vi "Periodic Tasks.vi"(8 "error in":errorcluster) -> ()   [LabVIEW 2014]
doc: "This VI runs in parallel to other tasks. It can contain as many user-defined periodic loops as you need. These can carry out PID or other sorts of timed response."
uses:
  <vilib>/Rock Robotics/WPI/Solenoid/WPI_SolenoidValue.ctl
  <vilib>/Rock Robotics/WPI/Joystick/WPI_JoystickGetSetRefNum.vi
  Robot Global Data.vi
  <vilib>/Rock Robotics/Network Tables/SD Write Boolean.vi
  <vilib>/Rock Robotics/Network Tables/SD Write Number.vi
  <vilib>/Rock Robotics/WPI/RobotDrive/WPI_RobotDriveGetSetRefNum.vi
  <vilib>/Rock Robotics/WPI/Solenoid/WPI_SolenoidSetEnum.vi
panel:
  out "pnumatics button 2":bool
  in  "Stopper Motor Speed Up":dbl(slide)=0.6 min=-1.0 max=1.0 step=0.05 scale=0.0..1.0 scale format="%#.3f"
  in  "Stopper Motor Speed Down":dbl(slide)=0.2 min=-1.0 max=1.0 step=0.05 scale=0.0..1.0 scale format="%#.3f"
  out "Actual Stopper Motor Speed":dbl
  out "Lifting Motor Speed Up":dbl
  out "Mode":bool
  out "Actual Lifting Motor Speed":dbl format="%#_13g"
  out "Trigger Switch Activated":bool=TRUE
  out "Upper Switch Activated":bool=TRUE
  out "Lower Switch Activated":bool=TRUE
  out "Accelerometer Chart":cluster{"X-Axis":dbl, "Y-Axis":dbl}(graph)
  out "X Acceleration":dbl format="%#_13g"
  out "Y Acceleration":dbl format="%#_13g"
  out "Degrees of Rotation":dbl format="%#_13g"
  out "pnumatics button":bool
  out "L":bool
  out "U":bool
  out "T":bool
  out "Running":bool
  out "Direction":bool
  in  "Lifting Motor Speed Down":dbl(slide)=0.39999999999999997 min=-1.0 max=1.0 step=0.05 scale=0.0..1.0 scale format="%#.3f"
  # "STOPPER\nMOTOR PANEL"
  # "GANTRY LIFT\nMOTOR PANEL"
  # "INDICATORS"
  # "LOGIC"
  # "CONTROLS"
  # "CONTROLS"
  # "INDICATORS"
  # "ACCELEROMETER\nPANEL"
  # "PNEUMATICS\nPANEL"
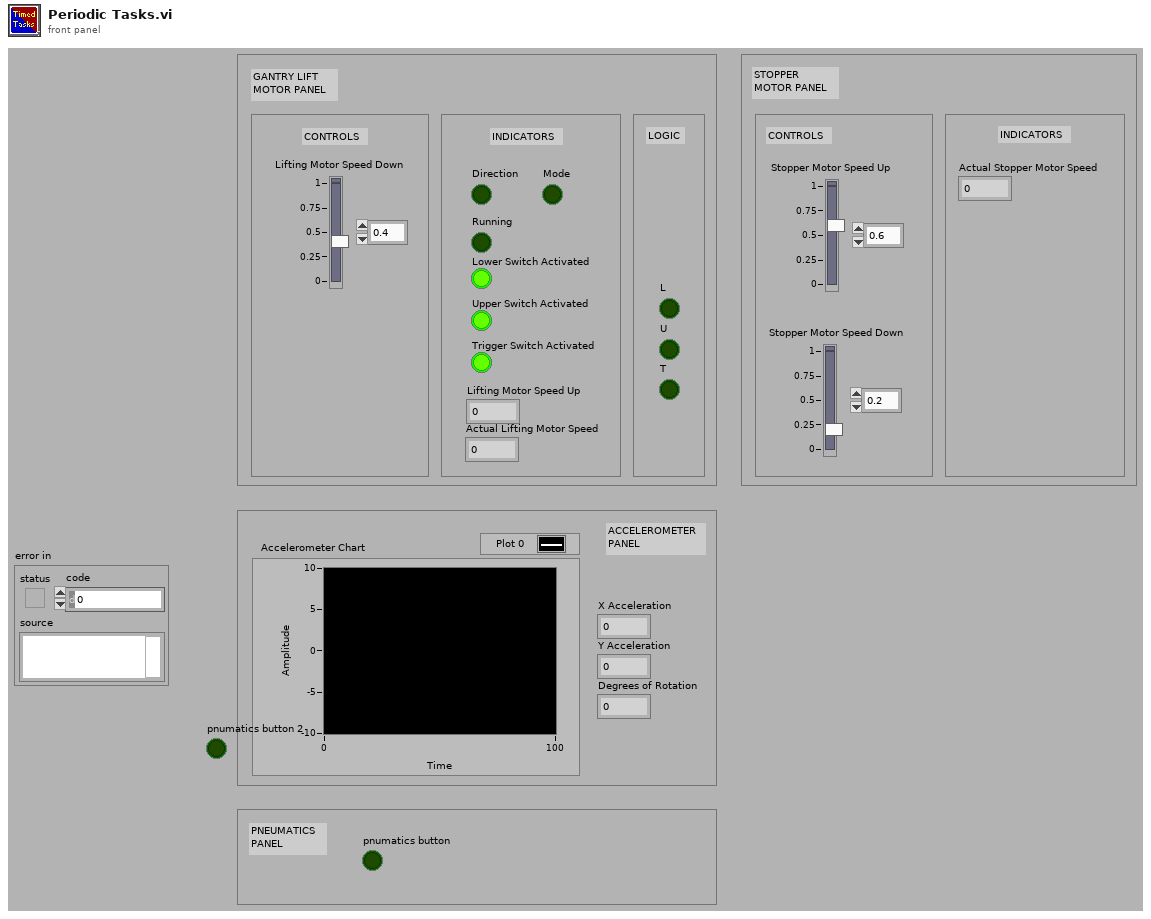
[diagram p1: front panel]
types:
  T1 = typedef "WPI_SolenoidValue.ctl" = enum16{"Off", "On", "Forward", "Reverse"}
  T2 = typedef "WPI_JoystickDevRef.ctl" = cluster{"Device":T3}
  T3 = typedef "WPI_JoystickDeviceEnum.ctl" = enum16{"USB 0", "USB 1", "USB 2", "USB 3", "USB 4", "USB 5"}
  T4 = typedef "WPI_SolenoidDevRef.ctl" = cluster{"DevStatus":errorcluster, "Pneumatics Control Module":u8, "Forward Solenoid Channel":T5, "Reverse Solenoid Channel":T5}
  T5 = typedef "WPI_SolenoidChannel.ctl" = enum8{"Solenoid 0", "Solenoid 1", "Solenoid 2", "Solenoid 3", "Solenoid 4", "Solenoid 5", "Solenoid 6", "Solenoid 7", "Invalid"}
  T6 = cluster{"JoystickDevRef":T2, "SolenoidDevRef":T4}
  T7 = typedef "WPI_AccelerometerDevRef.ctl" = cluster{"DevStatus":errorcluster, "Controller":T8, "Scaling":T9, "Analog Channels":T10, "I2C Bus":T12, "SPI Bus":T13, "Accel Range":T14, "ADXL345 Axes":T15, "Handle":i32, "Device Address":u8, "Accel Type":enum16{"Analog", "ADXL345 I2C", "ADXL345 SPI", "Internal"}}
  T8 = typedef "FPGA_TypedefAnalogModule.ctl" = enum16{"Controller 1"}
  T9 = typedef "WPI_AccelerometerScaling.ctl" = cluster{"Gain (VoltsPerG)":dbl, "Center Voltage":dbl}
  T10 = typedef "WPI_AccelerometerAnalogChannels.ctl" = cluster{"X-Axis":T11, "Y-Axis":T11, "Z-Axis":T11}
  T11 = typedef "FPGA_AIChannel.ctl" = enum8{"AI 0", "AI 1", "AI 2", "AI 3", "AI MXP 0", "AI MXP 1", "AI MXP 2", "AI MXP 3", "Invalid"}
  T12 = typedef "i2c_bus.ctl" = enum16{"I2C On-Board", "I2C MXP", "Invalid"}
  T13 = typedef "spi_bus.ctl" = enum16{"SPI On-Board, CS0", "SPI On-Board, CS1", "SPI On-Board, CS2", "SPI On-Board, CS3", "SPI MXP", "Invalid"}
  T14 = typedef "ADXL345 Range.ctl" = u8
  T15 = typedef "WPI_AccelerometerADXL345 Axes.ctl" = cluster{"X-Axis":bool, "Y-Axis":bool, "Z-Axis":bool}
  T16 = cluster{"X-Axis":dbl, "Y-Axis":dbl, "Z-Axis":dbl}
  T17 = typedef "WPI_MotorControlDeviceRef.ctl" = cluster{"DeviceStatus":errorcluster, "Type":T18, "PWM":cluster{"Controller":T19, "PWM Channel":T20, "DeadBand":T21}, "CAN":cluster{"Device Number":u8, "Control Mode":T22, "Semaphore":T23, "Max Vout":dbl, "TalonSRX Control Mode":T24}, "Invert":bool, "TransformRef":T25, "InvTransformRef":T25}
  T18 = typedef "WPI_MotorControlType.ctl" = enum16{"PWM", "CAN", "CANTalonSRX"}
  T19 = typedef "FPGA_TypedefDigitalModule.ctl" = enum16{"Controller 1"}
  T20 = typedef "FPGA_DIOPWMChannel.ctl" = enum8{"PWM 0", "PWM 1", "PWM 2", "PWM 3", "PWM 4", "PWM 5", "PWM 6", "PWM 7", "PWM 8", "PWM 9", "PWM MXP 0", "PWM MXP 1", "PWM MXP 2", "PWM MXP 3", "PWM MXP 4", "PWM MXP 5", "PWM MXP 6", "PWM MXP 7", "PWM MXP 8", "PWM MXP 9", "Invalid"}
  T21 = typedef "WPI_PWMDeadband.ctl" = cluster{"Name":string, "maxPositivePwm":i32, "minPositivePwm":i32, "centerPwm":i32, "maxNegativePwm":i32, "minNegativePwm":i32, "angularRange":u16}
  T22 = typedef "WPI_CANJaguar_ControlMode.ctl" = enum8{"Percent VBus", "Current", "Speed", "Position", "Voltage"}
  T23 = typedef "Semaphore RefNum" = refnum<k1>
  T24 = typedef "WPI_CANTalonSRX_APIControlMode.ctl" = enum8{"Percent VBus", "Speed", "Position", "Slave", "Unchanged / Invalid"}
  T25 = typedef "WPI_PWMTransform_ConPane.ctl" = refnum<vi>
  T26 = typedef "WPI_DigitalInputDevRef.ctl" = cluster{"DevStatus":errorcluster, "DIO Channel":T27, "Controller":T19}
  T27 = typedef "FPGA_DIOChannel.ctl" = enum8{"DIO 0", "DIO 1", "DIO 2", "DIO 3", "DIO 4", "DIO 5", "DIO 6", "DIO 7", "DIO 8", "DIO 9", "DIO MXP 0", "DIO MXP 1", "DIO MXP 2", "DIO MXP 3", "DIO MXP 4", "DIO MXP 5", "DIO MXP 6", "DIO MXP 7", "DIO MXP 8", "DIO MXP 9", "DIO MXP 10", "DIO MXP 11", "DIO MXP 12", "DIO MXP 13", "DIO MXP 14", "DIO MXP 15", "Invalid"}
  T28 = cluster{"JoystickDevRef":T2, "MotorControlDevRef":T17}
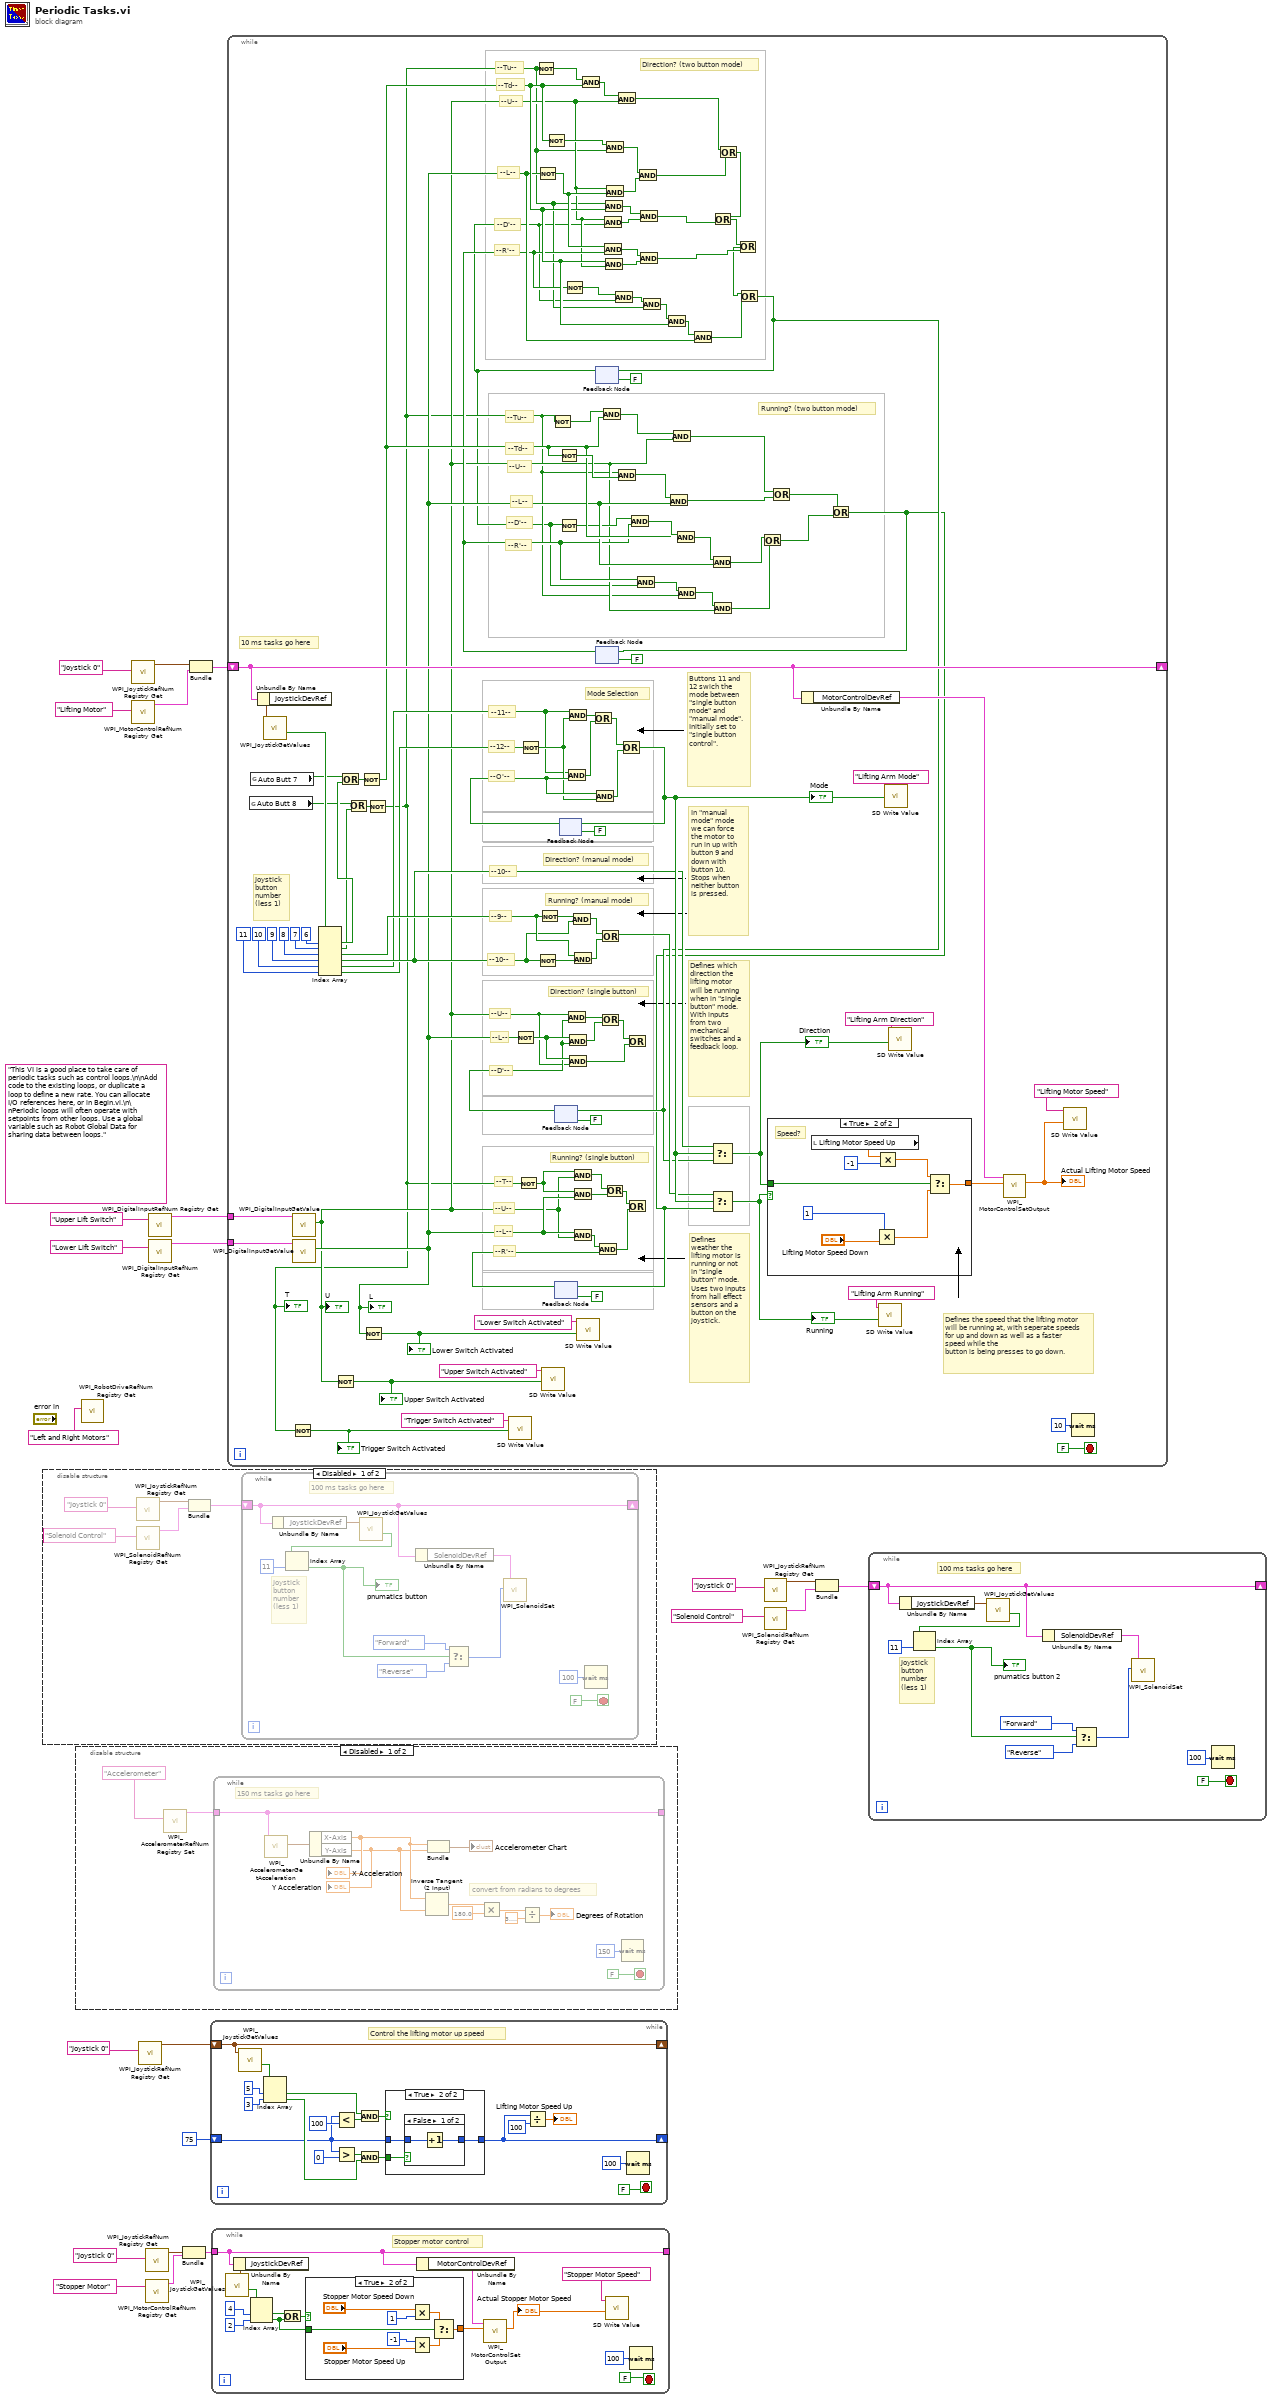
[diagram p0: block diagram]
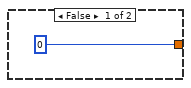
[diagram p2: hidden frame]
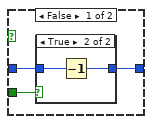
[diagram p3: hidden frame]
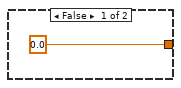
[diagram p8: hidden frame]
diagram:
  (unwired) "This VI is a good place to take care of periodic tasks such as control loops.\n\nAdd code to the existing loops, or duplicate a loop to define a new rate. You can allocate I/O references here, or in Begin.vi.\n\nPeriodic loops will often operate with setpoints from other loops. Use a global variable such as Robot Global Data for sharing data between loops."
  n1 = disable-structure shown="Disabled" {
    frame Disabled {
      n2 = call <vilib>:"WPI_JoystickRefNum Registry Get.vi"("refnum name"="Joystick 0") -> ("JoystickDevRef"=w26:T2)  [unwired: 1 in, 9 out]
      n3 = call <vilib>:"WPI_SolenoidRefNum Registry Get.vi"("refnum name"="Solenoid Control") -> ("SolenoidDevRef"=w25:T4)  [unwired: 9 in, 1 out]
      n4 = Bundle("JoystickDevRef"=w26, "SolenoidDevRef"=w25) -> (w24:T6)  [unwired: 1 out]
      n5 = while {
        shift-right: [w34] -> _
        shift-left: w24 -> [w34]
        stop <- FALSE stop-if-true
        # "Joystick button number (less 1)"
        # "100 ms tasks go here"
        n6 = Unbundle By Name(w34) -> ("JoystickDevRef"=w37:T2)
        n7 = call <vilib>:"WPI_JoystickGetValues.vi"("JoystickDevRef"=w37) -> ("Buttons"=w36:bool[])  [unwired: 6 in, 4 out]
        n8 = Index Array(array=w36, index=11) -> (element=w32:bool)
        "pnumatics button" <- w32
        n9 = Unbundle By Name(w34) -> ("SolenoidDevRef"=w33:T4)
        n10 = Select(t=WPI_SolenoidValue."Forward" ("Relay Value"), s=w32, f=WPI_SolenoidValue."Reverse" ("Relay Value")) -> (s? t:f=w29:T1)
        n11 = call-poly <vilib>:"WPI_SolenoidSet.vi"("Value"=w29, "SolenoidDevRef"=w33) -> ()  [unwired: 8 in, 2 out]
        n12 = Wait (ms)(milliseconds to wait=u32 100) -> ()  [unwired: 1 out]
      }
    }
    frame Enabled {
    }
  }
  n13 = disable-structure shown="Disabled" {
    frame Disabled {
      n14 = call <vilib>:"WPI_AccelerometerRefNum Registry Set.vi"("refnum name"="Accelerometer") -> ("AccelerometerDevRef"=w40:T7)  [unwired: 9 in, 1 out]
      n15 = while {
        tunnel: [w51] -> _
        tunnel: w40 -> [w51]
        stop <- FALSE stop-if-true
        # "convert from radians to degrees"
        # "150 ms tasks go here"
        n16 = call <vilib>:"WPI_AccelerometerGetAcceleration.vi"("AccelerometerDevRef"=w51) -> ("Accelerations"=w46:T16)  [unwired: 8 in, 2 out]
        n17 = Unbundle By Name(w46) -> ("X-Axis"=w44:dbl, "Y-Axis"=w43:dbl)
        "X Acceleration" <- w44
        "Y Acceleration" <- w43
        n18 = Inverse Tangent (2 Input)(1:w43, 2:w44) -> (0:w47:dbl)
        n19 = Bundle("X-Axis"=w44, "Y-Axis"=w43) -> (→"Accelerometer Chart":cluster{"X-Axis":dbl, "Y-Axis":dbl})  [unwired: 1 in]
        n20 = Multiply(x=w47, y=180.0) -> (x*y=w49:dbl)
        n21 = Divide(x=w49, y=3.141592653589793) -> (x/y=→"Degrees of Rotation":dbl)
        n22 = Wait (ms)(milliseconds to wait=u32 150) -> ()  [unwired: 1 out]
      }
    }
    frame Enabled {
    }
  }
  n23 = call <vilib>:"WPI_RobotDriveRefNum Registry Get.vi"("refnum name"="Left and Right Motors") -> ()  [unwired: 1 in, 10 out]
  n24 = call <vilib>:"WPI_JoystickRefNum Registry Get.vi"("refnum name"="Joystick 0") -> ("JoystickDevRef"=w19:T2)  [unwired: 1 in, 9 out]
  n25 = call <vilib>:"WPI_MotorControlRefNum Registry Get.vi"("refnum name"="Lifting Motor") -> ("MotorControlDevRef"=w15:T17)  [unwired: 9 in, 1 out]
  n26 = call <vilib>:"WPI_JoystickRefNum Registry Get.vi"("refnum name"="Joystick 0") -> ("JoystickDevRef"=w6:T2)  [unwired: 1 in, 9 out]
  n27 = call <vilib>:"WPI_JoystickRefNum Registry Get.vi"("refnum name"="Joystick 0") -> ("JoystickDevRef"=w10:T2)  [unwired: 1 in, 9 out]
  n28 = call <vilib>:"WPI_MotorControlRefNum Registry Get.vi"("refnum name"="Stopper Motor") -> ("MotorControlDevRef"=w9:T17)  [unwired: 9 in, 1 out]
  n29 = call <vilib>:"WPI_DigitalInputRefNum Registry Get.vi"("refnum name"="Upper Lift Switch") -> ("DigitalInputDevRef"=w17:T26)  [unwired: 9 in, 1 out]
  n30 = call <vilib>:"WPI_DigitalInputRefNum Registry Get.vi"("refnum name"="Lower Lift Switch") -> ("DigitalInputDevRef"=w16:T26)  [unwired: 9 in, 1 out]
  n31 = Bundle("JoystickDevRef"=w10, "MotorControlDevRef"=w9) -> (w8:T28)  [unwired: 1 in]
  n32 = Bundle("JoystickDevRef"=w19, "MotorControlDevRef"=w15) -> (w22:T28)  [unwired: 1 out]
  n33 = while {
    shift-right: [w64] -> _
    shift-left: 75 -> [w54]
    shift-right: [w56] -> _
    shift-left: w6 -> [w56]
    stop <- FALSE stop-if-true
    # "Control the lifting motor up speed"
    n34 = call <vilib>:"WPI_JoystickGetValues.vi"("JoystickDevRef"=w56) -> ("Buttons"=w62:bool[])  [unwired: 6 in, 4 out]
    n35 = Index Array(array=w62, index #1=5, index #2=3) -> (element #1=w59:bool, element #2=w58:bool)
    n36 = Less?(x=w54, y=100) -> (x < y?=w68:bool)
    n37 = Greater?(x=w54, y=0) -> (0:w67:bool)
    n38 = And(x=w59, y=w68) -> (x .and. y?=w66:bool)
    n39 = And(x=w67, y=w58) -> (x .and. y?=w65:bool)
    n40 = case shown="True" w66 {
      tunnel: w65 -> [w74 w80]
      tunnel: w54 -> [w73 w79]
      tunnel: [w72 w78] -> w64
      frame False {
        n41 = case shown="True" w74 {
          tunnel: w73 -> [w75 w77]
          tunnel: [w75 w76] -> w72
          frame False {
          }
          frame True {
            n42 = Decrement(x=w77) -> (x-1=w76:i32)
          }
        }
      }
      frame True {
        n43 = case shown="False" w80 {
          tunnel: w79 -> [w82 w83]
          tunnel: [w81 w83] -> w78
          frame False {
            n44 = Increment(x=w82) -> (x+1=w81:i32)
          }
          frame True {
          }
        }
      }
    }
    n45 = Divide(x=w64, y=100) -> (x/y=→"Lifting Motor Speed Up":dbl)
    n46 = Wait (ms)(milliseconds to wait=u32 100) -> ()  [unwired: 1 out]
  }
  n47 = while {
    tunnel: w8 -> [w88]
    tunnel: [w88] -> _
    stop <- FALSE stop-if-true
    # "Stopper motor control"
    n48 = Unbundle By Name(w88) -> ("JoystickDevRef"=w89:T2)
    n49 = call <vilib>:"WPI_JoystickGetValues.vi"("JoystickDevRef"=w89) -> ("Buttons"=w95:bool[])  [unwired: 6 in, 4 out]
    n50 = Index Array(array=w95, index #1=4, index #2=2) -> (element #1=w92:bool, element #2=w90:bool)
    n51 = Or(x=w92, y=w90) -> (x .or. y?=w91:bool)
    n52 = case shown="True" w91 {
      tunnel: w90 -> [_ w106]
      tunnel: [0 w104] -> w86
      frame False {
      }
      frame True {
        n53 = Multiply(x="Stopper Motor Speed Down", y=1) -> (x*y=w105:dbl)
        n54 = Multiply(x=-1, y="Stopper Motor Speed Up") -> (x*y=w101:dbl)
        n55 = Select(t=w105, s=w106, f=w101) -> (s? t:f=w104:dbl)
      }
    }
    n56 = Unbundle By Name(w88) -> ("MotorControlDevRef"=w87:T17)
    n57 = call <vilib>:"WPI_MotorControlSetOutput.vi"("Output"=w86, "MotorControlDevRef"=w87) -> ("Motor Output"=w84:dbl)  [unwired: 7 in, 2 out]
    "Actual Stopper Motor Speed" <- w84
    n58 = call-poly <vilib>:"SD Write Value.vi"("Numeric"=w84, "Name"="Stopper Motor Speed" ("refnum name")) -> ()  [unwired: 8 in, 2 out]
    n59 = Wait (ms)(milliseconds to wait=u32 100) -> ()  [unwired: 1 out]
  }
  n60 = while {
    shift-right: [w213] -> _
    shift-left: w22 -> [w213]
    tunnel: w17 -> [w217]
    tunnel: w16 -> [w215]
    stop <- FALSE stop-if-true
    # "Running? (two button mode)"
    # "Direction? (two button mode)"
    # "--R'--"
    # "--D'--"
    # "--L--"
    # "--U--"
    # "--Td--"
    # "--Tu--"
    # "--D'--"
    # "--R'--"
    # "--L--"
    # "--U--"
    # "--Td--"
    # "--Tu--"
    # "--10--"
    # "Direction? (manual mode)"
    # "--R'--"
    # "Running? (manual mode)"
    # "--O'--"
    # "Defines the speed that the lifting motor will be running at, with seperate speeds for up and down as well as a faster speed while the \nbutton is being presses to go down."
    # "Defines weather the lifting motor is running or not in \"single button\" mode. Uses two inputs from hall effect sensors and a button on the joystick."
    # "Defines which direction the lifting motor will be running when in \"single button\" mode. With inputs from two mechanical switches and a feedback loop."
    # "In \"manual mode\" mode we can force the motor to run in up with button 9 and down with button 10. Stops when neither button is pressed."
    # "Buttons 11 and 12 swich the mode between  \"single button mode\" and \"manual mode\". Initially set to \"single button control\"."
    # "--12--"
    # "--11--"
    # "--10--"
    # "--9--"
    # "Mode Selection"
    # "Joystick button number (less 1)"
    # "--U--"
    # "--L--"
    # "--T--"
    # "--D'--"
    # "--U--"
    # "--L--"
    # "Direction? (single button)"
    # "Running? (single button)"
    # "10 ms tasks go here"
    n61 = global read "Robot Global Data.vi" "Auto Butt 8"() -> (w109:bool)
    n62 = global read "Robot Global Data.vi" "Auto Butt 7"() -> (w113:bool)
    n63 = Unbundle By Name(w213) -> ("JoystickDevRef"=w216:T2)
    n64 = call <vilib>:"WPI_JoystickGetValues.vi"("JoystickDevRef"=w216) -> ("Buttons"=w195:bool[])  [unwired: 6 in, 4 out]
    n65 = call <vilib>:"WPI_DigitalInputGetValue.vi"("DigitalInputDevRef"=w217) -> ("Value"=w125:bool)  [unwired: 8 in, 2 out]
    "U" <- w125
    n66 = call <vilib>:"WPI_DigitalInputGetValue.vi"("DigitalInputDevRef"=w215) -> ("Value"=w131:bool)  [unwired: 8 in, 2 out]
    "L" <- w131
    n67 = Index Array(array=w195, index #1=u32 6 ("milliseconds to wait"), index #2=u32 7 ("milliseconds to wait"), index #3=u32 8 ("milliseconds to wait"), index #4=u32 9 ("milliseconds to wait"), index #5=u32 10 ("milliseconds to wait"), index #6=u32 11 ("milliseconds to wait")) -> (element #1=w112:bool, element #2=w110:bool, element #3=w170:bool, element #4=w166:bool, element #5=w163:bool, element #6=w162:bool)
    n68 = Not(x=w125) -> (.not. x?=w202:bool)
    "Upper Switch Activated" <- w202
    n69 = Or(x=w113, y=w112) -> (x .or. y?=w111:bool)
    n70 = Or(x=w109, y=w110) -> (x .or. y?=w197:bool)
    n71 = Not(x=w111) -> (.not. x?=w133:bool)
    n72 = Not(x=w131) -> (.not. x?=w203:bool)
    "Lower Switch Activated" <- w203
    n73 = Not(x=w197) -> (.not. x?=w124:bool)
    "T" <- w124
    n74 = Not(x=w124) -> (.not. x?=w200:bool)
    "Trigger Switch Activated" <- w200
    n75 = call-poly <vilib>:"SD Write Value.vi"("Boolean"=w200, "Name"="Trigger Switch Activated" ("refnum name")) -> ()  [unwired: 8 in, 2 out]
    n76 = Not(x=w131) -> (.not. x?=w183:bool)
    n77 = Not(x=w124) -> (.not. x?=w186:bool)
    n78 = Not(x=w162) -> (.not. x?=w177:bool)
    n79 = Not(x=w124) -> (.not. x?=w160:bool)
    n80 = Not(x=w131) -> (.not. x?=w139:bool)
    n81 = Not(x=w166) -> (.not. x?=w171:bool)
    n82 = Not(x=w170) -> (.not. x?=w172:bool)
    n83 = call-poly <vilib>:"SD Write Value.vi"("Boolean"=w202, "Name"="Upper Switch Activated" ("refnum name")) -> ()  [unwired: 8 in, 2 out]
    n84 = Not(x=w133) -> (.not. x?=w157:bool)
    n85 = Not(x=w124) -> (.not. x?=w126:bool)
    n86 = feedback #1(FALSE) -> (w178:bool)
    n87 = feedback #2(FALSE) -> (w185:bool)
    n88 = Not(x=w133) -> (.not. x?=w135:bool)
    n89 = feedback #3(FALSE) -> (w190:bool)
    n90 = And(x=w163, y=w190) -> (x .and. y?=w193:bool)
    n91 = And(x=w125, y=w178) -> (x .and. y?=w181:bool)
    n92 = And(x=w163, y=w177) -> (x .and. y?=w194:bool)
    n93 = And(x=w183, y=w178) -> (x .and. y?=w180:bool)
    n94 = And(x=w183, y=w125) -> (x .and. y?=w179:bool)
    n95 = And(x=w172, y=w166) -> (x .and. y?=w169:bool)
    n96 = And(x=w170, y=w171) -> (x .and. y?=w168:bool)
    n97 = And(x=w186, y=w125) -> (x .and. y?=w208:bool)
    n98 = And(x=w186, y=w131) -> (x .and. y?=w207:bool)
    n99 = And(x=w131, y=w125) -> (x .and. y?=w187:bool)
    n100 = call-poly <vilib>:"SD Write Value.vi"("Boolean"=w203, "Name"="Lower Switch Activated" ("refnum name")) -> ()  [unwired: 8 in, 2 out]
    n101 = And(x=w160, y=w133) -> (x .and. y?=w158:bool)
    n102 = Or(x=w194, y=w193) -> (x .or. y?=w192:bool)
    n103 = And(x=w190, y=w177) -> (x .and. y?=w191:bool)
    n104 = feedback #4(FALSE) -> (w123:bool)
    n105 = Not(x=w123) -> (.not. x?=w127:bool)
    n106 = feedback #5(FALSE) -> (w128:bool)
    n107 = Not(x=w128) -> (.not. x?=w138:bool)
    n108 = And(x=w187, y=w185) -> (x .and. y?=w184:bool)
    n109 = Or(x=w169, y=w168) -> (x .or. y?=w167:bool)
    n110 = Or(x=w181, y=w180) -> (x .or. y?=w182:bool)
    n111 = And(x=w126, y=w133) -> (x .and. y?=w137:bool)
    n112 = And(x=w125, y=w123) -> (x .and. y?=w151:bool)
    n113 = And(x=w139, y=w128) -> (x .and. y?=w148:bool)
    n114 = And(x=w124, y=w133) -> (x .and. y?=w152:bool)
    n115 = And(x=w133, y=w125) -> (x .and. y?=w147:bool)
    n116 = And(x=w157, y=w124) -> (x .and. y?=w156:bool)
    n117 = And(x=w125, y=w139) -> (x .and. y?=w155:bool)
    n118 = Or(x=w208, y=w207) -> (x .or. y?=w206:bool)
    n119 = And(x=w138, y=w123) -> (x .and. y?=w144:bool)
    n120 = And(x=w158, y=w125) -> (x .and. y?=w116:bool)
    n121 = And(x=w124, y=w135) -> (x .and. y?=w136:bool)
    n122 = Or(x=w192, y=w191) -> (x .or. y?=w175:bool)
    "Mode" <- w175
    n123 = feedback-in #3(w175) -> ()
    n124 = Or(x=w182, y=w179) -> ()  [unwired: 1 out]
    n125 = Or(x=w206, y=w184) -> ()  [unwired: 1 out]
    n126 = And(x=w127, y=w128) -> (x .and. y?=w134:bool)
    n127 = And(x=w128, y=w123) -> (x .and. y?=w129:bool)
    n128 = And(x=w156, y=w155) -> (x .and. y?=w154:bool)
    n129 = And(x=w152, y=w151) -> (x .and. y?=w150:bool)
    n130 = And(x=w148, y=w147) -> (x .and. y?=w146:bool)
    n131 = And(x=w144, y=w124) -> (x .and. y?=w143:bool)
    n132 = And(x=w143, y=w133) -> (x .and. y?=w142:bool)
    n133 = And(x=w136, y=w131) -> (x .and. y?=w121:bool)
    n134 = And(x=w137, y=w125) -> (x .and. y?=w122:bool)
    n135 = And(x=w134, y=w133) -> (x .and. y?=w132:bool)
    n136 = And(x=w129, y=w124) -> (x .and. y?=w130:bool)
    n137 = And(x=w142, y=w131) -> (x .and. y?=w140:bool)
    n138 = And(x=w132, y=w131) -> (x .and. y?=w120:bool)
    n139 = And(x=w130, y=w125) -> (x .and. y?=w119:bool)
    n140 = Or(x=w116, y=w154) -> (x .or. y?=w161:bool)
    n141 = Or(x=w161, y=w150) -> (x .or. y?=w145:bool)
    n142 = Or(x=w145, y=w146) -> (x .or. y?=w141:bool)
    n143 = Or(x=w141, y=w140) -> (x .or. y?=w115:bool)
    n144 = feedback-in #1(w115) -> ()
    n145 = feedback-in #4(w115) -> ()
    n146 = Select(t=w166, s=w175, f=w115) -> (s? t:f=w174:bool)
    "Direction" <- w174
    n147 = Or(x=w120, y=w119) -> (x .or. y?=w117:bool)
    n148 = Or(x=w122, y=w121) -> (x .or. y?=w118:bool)
    n149 = Unbundle By Name(w213) -> ("MotorControlDevRef"=w212:T17)
    n150 = Or(x=w118, y=w117) -> (x .or. y?=w114:bool)
    n151 = feedback-in #2(w114) -> ()
    n152 = feedback-in #5(w114) -> ()
    n153 = Select(t=w167, s=w175, f=w114) -> (s? t:f=w173:bool)
    "Running" <- w173
    n154 = case shown="True" w173 {
      tunnel: w174 -> [_ w228]
      tunnel: [0.0 ("Throw Motor Speed (-1 to 1) 2") w227] -> w198
      frame False {
      }
      frame True {
        # "Speed?"
        n155 = local read "Lifting Motor Speed Up"() -> (w221:dbl)
        n156 = Multiply(x=1, y="Lifting Motor Speed Down") -> (x*y=w224:dbl)
        n157 = Multiply(x=w221, y=-1) -> (x*y=w225:dbl)
        n158 = Select(t=w225, s=w228, f=w224) -> (s? t:f=w227:dbl)
      }
    }
    n159 = call-poly <vilib>:"SD Write Value.vi"("Boolean"=w173, "Name"="Lifting Arm Running" ("refnum name")) -> ()  [unwired: 8 in, 2 out]
    n160 = call-poly <vilib>:"SD Write Value.vi"("Boolean"=w175, "Name"="Lifting Arm Mode" ("refnum name")) -> ()  [unwired: 8 in, 2 out]
    n161 = call-poly <vilib>:"SD Write Value.vi"("Boolean"=w174, "Name"="Lifting Arm Direction" ("refnum name")) -> ()  [unwired: 8 in, 2 out]
    n162 = call <vilib>:"WPI_MotorControlSetOutput.vi"("Output"=w198, "MotorControlDevRef"=w212) -> ("Motor Output"=w108:dbl)  [unwired: 7 in, 2 out]
    "Actual Lifting Motor Speed" <- w108
    n163 = call-poly <vilib>:"SD Write Value.vi"("Numeric"=w108, "Name"="Lifting Motor Speed" ("refnum name")) -> ()  [unwired: 8 in, 2 out]
    n164 = Wait (ms)(milliseconds to wait=u32 10) -> ()  [unwired: 1 out]
  }
  n165 = call <vilib>:"WPI_JoystickRefNum Registry Get.vi"("refnum name"="Joystick 0") -> ("JoystickDevRef"=w3:T2)  [unwired: 1 in, 9 out]
  n166 = call <vilib>:"WPI_SolenoidRefNum Registry Get.vi"("refnum name"="Solenoid Control") -> ("SolenoidDevRef"=w2:T4)  [unwired: 9 in, 1 out]
  n167 = Bundle("JoystickDevRef"=w3, "SolenoidDevRef"=w2) -> (w1:T6)  [unwired: 1 out]
  n168 = while {
    shift-right: [w234] -> _
    shift-left: w1 -> [w234]
    stop <- FALSE stop-if-true
    # "Joystick button number (less 1)"
    # "100 ms tasks go here"
    n169 = Unbundle By Name(w234) -> ("JoystickDevRef"=w237:T2)
    n170 = call <vilib>:"WPI_JoystickGetValues.vi"("JoystickDevRef"=w237) -> ("Buttons"=w236:bool[])  [unwired: 6 in, 4 out]
    n171 = Index Array(array=w236, index=11) -> (element=w232:bool)
    "pnumatics button 2" <- w232
    n172 = Unbundle By Name(w234) -> ("SolenoidDevRef"=w233:T4)
    n173 = Select(t=WPI_SolenoidValue."Forward" ("Relay Value"), s=w232, f=WPI_SolenoidValue."Reverse" ("Relay Value")) -> (s? t:f=w229:T1)
    n174 = call-poly <vilib>:"WPI_SolenoidSet.vi"("Value"=w229, "SolenoidDevRef"=w233) -> ()  [unwired: 8 in, 2 out]
    n175 = Wait (ms)(milliseconds to wait=u32 100) -> ()  [unwired: 1 out]
  }
